vi "3D_Scatter_Plot_ph.vi"(11 "XYUVArray":dbl[][](array[numeric])=[[-138.0, 28.0, -5.0, -3.0], [-92.0, 28.0, -10.0, -5.5], [-46.0, 28.0, -5.0, -10.5], [0.0, 28.0, -9.0, 3.5], [46.0, 28.0, -22.0, 1.0], [92.0, 28.0, -24.5, -9.0], [138.0, 28.0, -16.0, -23.0], [-138.0, 60.0, -6.0, -2.0], [-92.0, 60.0, -7.0, -12.0], [-46.0, 60.0, -6.0, -11.0], [0.0, 60.0, -9.0, 3.0], [46.0, 60.0, -5.5, 6.0], [92.0, 60.0, -10.0, -7.5], [138.0, 60.0, -17.0, -22.0], [-138.0, 92.0, 0.5, 2.0], [-92.0, 92.0, -1.5, -15.0], [-46.0, 92.0, -1.5, -10.5], [0.0, 92.0, 1.0, -1.5], [46.0, 92.0, 1.0, 3.0], [92.0, 92.0, -2.5, -7.5], [138.0, 92.0, -5.0, -17.0], [-138.0, 124.0, 18.5, 15.0], [-92.0, 124.0, 10.5, -2.5], [-46.0, 124.0, 6.5, -2.0], [0.0, 124.0, 7.5, 5.0], [46.0, 124.0, 9.5, 12.5], [92.0, 124.0, 14.0, 8.5], [138.0, 124.0, 6.5, -4.0], [-138.0, 156.0, 13.5, 14.5], [-92.0, 156.0, 19.5, 4.0], [-46.0, 156.0, 12.5, -1.0], [0.0, 156.0, 10.5, 3.5], [46.0, 156.0, 14.0, 11.0], [92.0, 156.0, 17.5, 10.5], [138.0, 156.0, 12.0, -4.5], [-138.0, 188.0, 9.0, 16.5], [-92.0, 188.0, 10.0, 8.0], [-46.0, 188.0, 14.0, 4.0], [0.0, 188.0, 15.5, 8.0], [46.0, 188.0, 14.5, 11.0], [92.0, 188.0, 21.5, 11.0], [138.0, 188.0, 19.0, 0.5], [-138.0, 214.0, 12.5, 11.5], [-92.0, 214.0, 17.5, 6.0], [-46.0, 214.0, 17.0, 9.5], [0.0, 214.0, 14.5, 10.5], [46.0, 214.0, 19.0, 10.5], [92.0, 214.0, 20.0, 7.0], [138.0, 214.0, 16.5, 7.0]]) -> ()   [LabVIEW 2011]
uses:
  <vilib>/Math Plots/3D Math Plots/3D Scatter/3D Scatter XCtrl/3D Scatter.xctl
  <vilib>/Math Plots/3D Math Plots/3D Scatter/3D Scatter Datatype/Public/Plot Helper (Vector).vi
  <vilib>/Math Plots/3D Math Plots/3D Scatter/3D Scatter Datatype/3D Scatter Datatype.lvclass
panel:
  out "3D Scatter":refnum<class "3D Plot Datatype.lvclass">[](xcontrol)
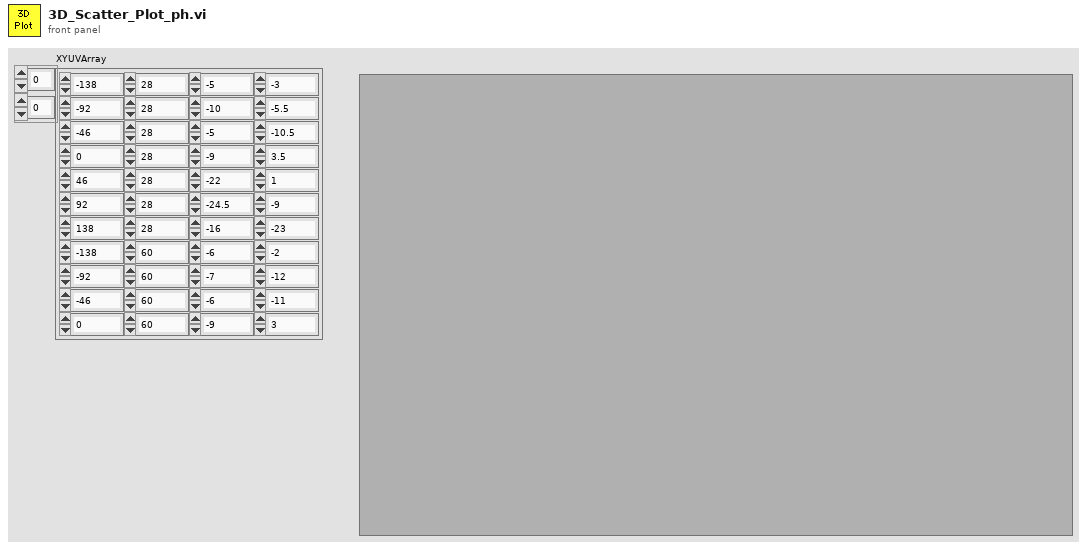
[diagram p1: front panel]
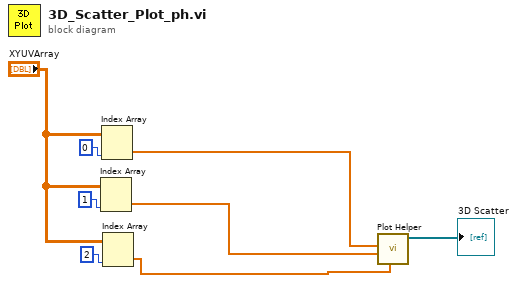
[diagram p0: block diagram]
diagram:
  n1 = Index Array(array="XYUVArray", index (col)=1 ("index (row)")) -> (element=w2:dbl[])  [unwired: 1 in]
  n2 = Index Array(array="XYUVArray", index (col)=0 ("index (row)")) -> (element=w1:dbl[])  [unwired: 1 in]
  n3 = Index Array(array="XYUVArray", index (col)=2 ("index (row)")) -> (element=w4:dbl[])  [unwired: 1 in]
  n4 = call-poly <vilib>:"Plot Helper.vi"("z vector"=w4, "y vector"=w2, "x vector"=w1) -> ("3D Plot lvclass Array out"=→"3D Scatter":refnum<class "3D Plot Datatype.lvclass">[])  [unwired: 3 in, 5 out]
